vi "txt.vi"(0 "file name":string="measure", 9 "array":dbl[][](array[numeric]), 11 "error in":errorcluster) -> (4 "acquired data":cluster{dbl[], dbl[]}(graph), 8 "output cluster":T1, 10 "mean":dbl, 15 "error out":errorcluster)   [LabVIEW 2014]
uses:
  <vilib>/Analysis/NI_AALBase.lvlib
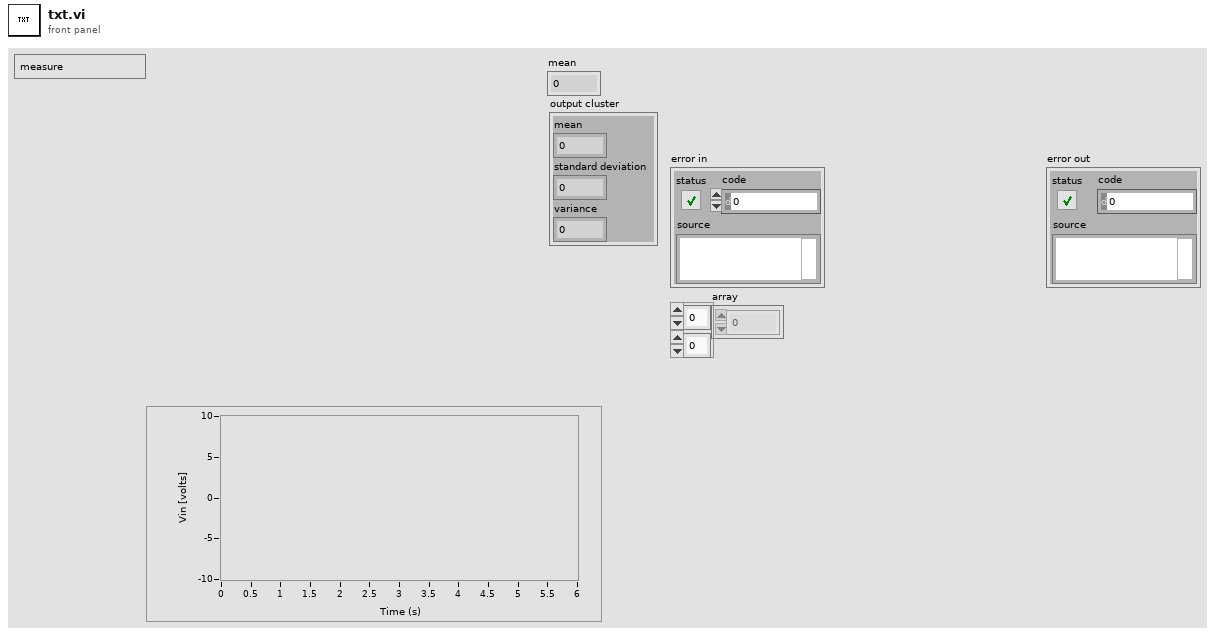
[diagram p1: front panel]
types:
  T1 = cluster{"mean":dbl, "standard deviation":dbl, "variance":dbl}
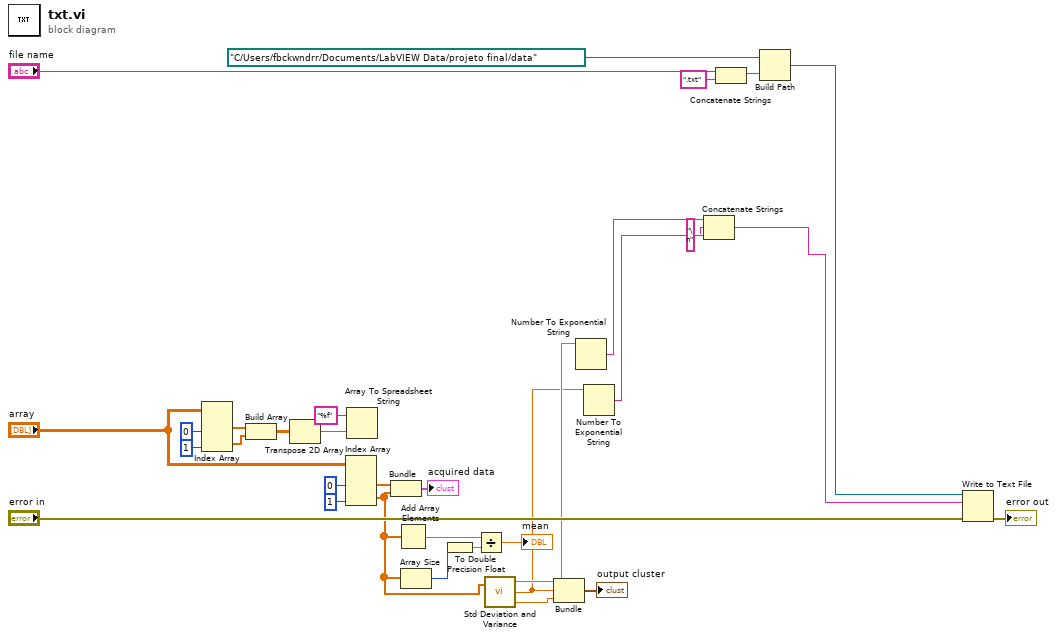
[diagram p0: block diagram]
diagram:
  n1 = Index Array(array="array", index (col) #1=0 ("disabled index (col)"), index (col) #2=1 ("index (col)")) -> (element #1=w24:dbl[], element #2=w23:dbl[])  [unwired: 2 in]
  n2 = Build Array(w24, w23) -> (w25:dbl[][])
  n3 = Transpose 2D Array(2D array=w25) -> (transposed array=w22:dbl[][])
  n4 = Index Array(array="array", index (col) #1=0 ("disabled index (col)"), index (col) #2=1 ("index (col)")) -> (element #1=w29:dbl[], element #2=w8:dbl[])  [unwired: 2 in]
  n5 = Array To Spreadsheet String(array=w22, 3:"%f" ("format string")) -> ()  [unwired: 1 in, 1 out]
  n6 = Bundle("array"=w29, "array"=w8) -> (→"acquired data":cluster{"array":dbl[], "array":dbl[]})  [unwired: 1 in]
  n7 = Add Array Elements(numeric array=w8) -> (sum=w12:dbl)
  n8 = Array Size(array=w8) -> (size(s)=w11:i32)
  n9 = To Double Precision Float(number=w11) -> (double precision float=w10:dbl)
  n10 = Divide(x=w12, y=w10) -> (x/y=→"mean":dbl)
  n11 = call <vilib>:"Std Deviation and Variance.vi"("X"=w8) -> ("mean"=w5:dbl, "standard deviation"=w4:dbl, "variance"=w7:dbl)  [unwired: 1 in]
  n12 = Bundle("mean"=w5, "standard deviation"=w4, "variance"=w7) -> (→"output cluster":T1)  [unwired: 1 in]
  n13 = Number To Exponential String(number=w5) -> (E-format string=w3:string)  [unwired: 3 in]
  n14 = Number To Exponential String(number=w4) -> (E-format string=w2:string)  [unwired: 3 in]
  n15 = Concatenate Strings(w3, "\n" ("string"), w2) -> (w17:string)
  n16 = Concatenate Strings("file name", ".txt" ("string")) -> (w20:string)
  n17 = Build Path(base path=path "C:/Users/fbckwndrr/Documents/LabVIEW Data/projeto final/data", name or relative path=w20) -> (appended path=w16:path)
  n18 = Write to Text File(file (use dialog)=w16, text=w17, error in="error in") -> (error out=→"error out":errorcluster)  [unwired: 1 in, 2 out]
